vi "test_BuildEvalStr_Int_Equal.vi"(8 "error in (no error)":errorcluster, 11 "TestCase in":refnum<class "Build Eval Str Test Case.lvclass">) -> (0 "error out":errorcluster, 3 "TestCase out":refnum<class "Build Eval Str Test Case.lvclass">)   [LabVIEW 2018, in "Build Eval Str Test Case.lvclass"]
uses:
  Build Eval Str Test Case.lvclass
  Plugins/Utility/Test Classes/Integer/Equal/Int Equal.lvclass
  C:/Users/UKHornP/Documents/Work/Projects/Assert API/Plugins/Utility/Test Classes/Test.lvclass
  Plugins/Utility/Test Classes/Test Class String IDs.vi
  <vilib>/addons/_JKI Toolkits/VI Tester/TestCase.llb/TestCase.lvclass
  Plugins/Utility/Test Classes/Test.lvclass
  C:/Program Files (x86)/National Instruments/LabVIEW 2018/vi.lib/addons/_JKI Toolkits/VI Tester/TestCase.llb/TestCase.lvclass
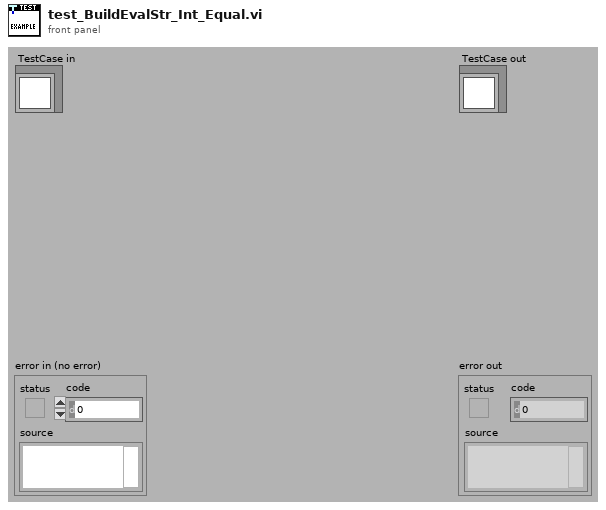
[diagram p1: front panel]
types:
  T1 = cluster{"Comparison Value 1":string, "Comparison Value 2":string, "Invert Result":string, "Assert VI Name":string, "Data Type":string, "Builder User Name":string, "Build Timestamp":string, "Failure Action":string, "Comment":string, "Assert Name":string, "Description":string, "Evaluation String":string}
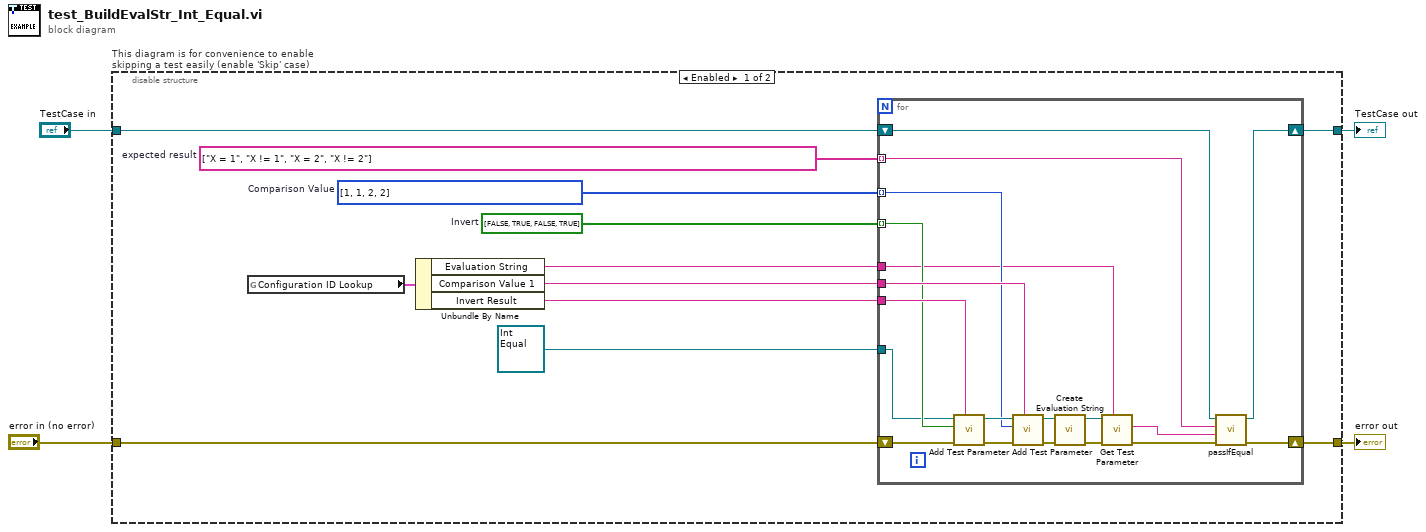
[diagram p0: block diagram]
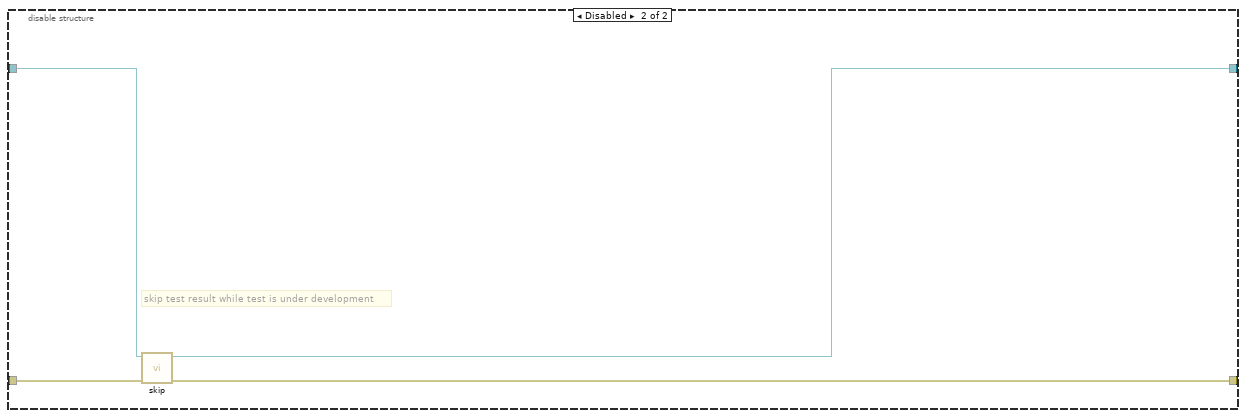
[diagram p2: hidden frame]
diagram:
  n1 = disable-structure "This diagram is for convenience to enable skipping a test easily (enable 'Skip' case)" shown="Enabled" {
    disable-tunnel: "TestCase in" -> [w15 w39]
    disable-tunnel: [w14 w37] -> w1
    disable-tunnel: [w13 w38] -> w3
    disable-tunnel: "error in (no error)" -> [w6 w36]
    frame Enabled {
      w7 = i32[] [1, 1, 2, 2]  # Comparison Value
      w8 = bool[] [FALSE, TRUE, FALSE, TRUE]  # Invert
      w16 = string[] ["X = 1", "X != 1", "X = 2", "X != 2"]  # expected result
      n2 = global read "Test Class String IDs.vi" "Configuration ID Lookup"() -> (w11:T1)
      n3 = Unbundle By Name(w11) -> ("Evaluation String"=w5:string, "Comparison Value 1"=w9:string, "Invert Result"=w10:string)
      n4 = for {
        tunnel: w16 -> [w35] mode=indexing
        tunnel: refnum<class "Int Equal.lvclass"> refnum ("Int Equal.lvclass") -> [w17]
        tunnel: w10 -> [w31]
        tunnel: w9 -> [w30]
        tunnel: w8 -> [w28] mode=indexing
        tunnel: w7 -> [w27] mode=indexing
        tunnel: w5 -> [w19]
        shift-right: [w33] -> w14
        shift-left: w15 -> [w34]
        shift-right: [w32] -> w13
        shift-left: w6 -> [w26]
        n5 = call-dynamic "Add Test Parameter.vi"("Data Value ID"=w31, "error in (no error)"=w26, "Data Value"=w28, "Test in"=w17) -> ("error out"=w25:errorcluster, "Test out"=w29:refnum<class "Int Equal.lvclass">)  [unwired: 5 in, 1 out]
        n6 = call-dynamic "Add Test Parameter.vi"("Data Value ID"=w30, "error in (no error)"=w25, "Data Value"=w27, "Test in"=w29) -> ("error out"=w23:errorcluster, "Test out"=w24:refnum<class "Int Equal.lvclass">)  [unwired: 5 in, 1 out]
        n7 = call-dynamic "Create Evaluation String.vi"("error in (no error)"=w23, "Int Equal in"=w24) -> ("error out"=w22:errorcluster, "Int Equal out"=w20:refnum<class "Int Equal.lvclass">)  [unwired: 8 in]
        n8 = call "Get Test Parameter.vi"("Data Value ID"=w19, "error in (no error)"=w22, "Test in"=w20) -> ("error out"=w21:errorcluster, "Test Parameter"=w18:string)  [unwired: 6 in, 1 out]
        n9 = call-dynamic "passIfEqual.vi"("error in (no error)"=w21, "y"=w18, "x"=w35, "TestCase in"=w34) -> ("error out"=w32:errorcluster, "TestCase out"=w33:refnum<class "Build Eval Str Test Case.lvclass">)  [unwired: 6 in]
      }
    }
    frame Disabled {
      # "skip test result while test is under development"
      n10 = call <vilib>:"skip.vi"("error in (no error)"=w36, "TestCase in"=w39) -> ("error out"=w38:errorcluster, "TestCase out"=w37:refnum<class "Build Eval Str Test Case.lvclass">)  [unwired: 8 in]
    }
  }
  "error out" <- w3
  "TestCase out" <- w1
